vi "Scan Abort.vi"(8 "error in (no error)":errorcluster, 10 "Reference to a Stop button":refnum<vi>, 11 "VISA resource name":refnum<visa-resource-name>) -> (0 "error out":errorcluster, 3 "VISA resource name out":refnum<visa-resource-name>)   [LabVIEW 2009, in "Digikrom DK24x.lvlib"]
doc: "Inner loop that waits until scan completes or user pushes a specified abort button. Sends cancel command and stops all movement."
uses:
  Digikrom DK24x.lvlib
  Command.ctl
panel:
  in  "Manual Abort":bool
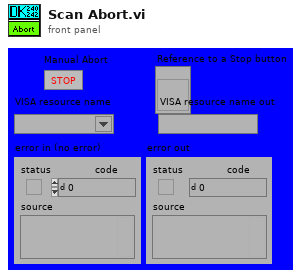
[diagram p1: front panel]
types:
  T1 = typedef "Digikrom DK24x.lvlib/Command.ctl" = u8
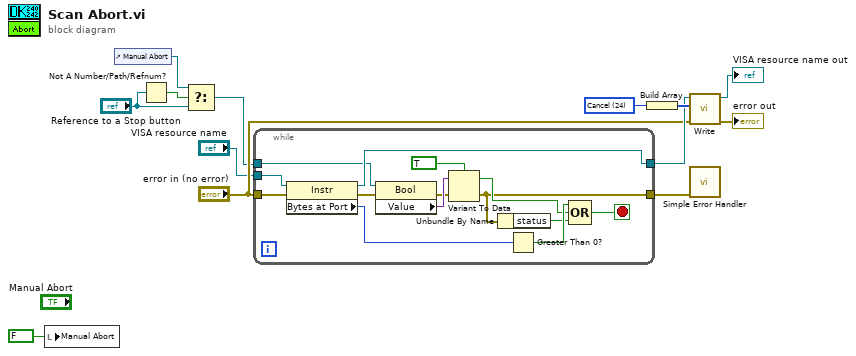
[diagram p0: block diagram]
diagram:
  w1 = T1 24 items=["Cancel"=24, "Clear"=25, "CSR"=28, "Echo"=27, "Filter"=15, "Gcal"=18, "Goto"=16, "Grtid?"=19, "Grtsel"=26, "NOVRAM Read"=56, "NOVRAM Write"=59, "Reset"=255, "Scan"=12, "Scan Up"=9, "Scan Down"=3, "Serial?"=33, "Slew Up"=8, "Slew Down"=2, "Slit Reset"=43, "Slit?"=30, "Sltadj"=14, "Speed"=13, "Sspeed?"=21, "Step Down"=1, "Step Up"=7, "S1adj"=31, "S2adj"=32, "S3adj"=34, "S1cal"=22, "S2cal"=23, "S3cal"=35, "Test"=17, "Type"=57, "Wave?"=29, "Zero"=52] ("Command")
  n1 = local write "Manual Abort"(FALSE ("Manual Abort")) -> ()
  n2 = control-ref of="Manual Abort"() -> (w6:refnum<vi>)
  n3 = Not A Number/Path/Refnum?(number/path/refnum="Reference to a Stop button") -> (NaN/Path/Refnum?=w4:bool)
  n4 = Select(t=w6, s=w4, f="Reference to a Stop button") -> (s? t:f=w3:refnum<vi>)
  n5 = while {
    tunnel: "error in (no error)" -> [w27]
    tunnel: "VISA resource name" -> [w25]
    tunnel: [w24] -> w12
    tunnel: [w16] -> w8
    tunnel: w3 -> [w14]
    stop <- w22 stop-if-true
    n6 = property class="Instr"(reference=w25, error in=w27) -> (reference out=w24:refnum<visa-resource-name>, error out=w26:errorcluster, "Bytes at Port"=w23:u32)
    n7 = property class="Bool"(reference=w14, error in=w26) -> (error out=w19:errorcluster, "Value"=w21:variant)  [unwired: 1 out]
    n8 = Variant To Data(error in=w19, Variant=w21, type=TRUE) -> (error out=w16:errorcluster, data=w17:bool)
    n9 = Unbundle By Name(w16) -> ("status"=w15:bool)
    n10 = Greater Than 0?(x=w23) -> (x > 0?=w18:bool)
    n11 = Compound Arithmetic op=OR(w18, w17, w15) -> (w22:bool)
  }
  n12 = Build Array(w1) -> (w13:T1[])
  n13 = call "Write.vi"("error in (no error)"="error in (no error)", "Byte Array"=w13, "VISA resource name"=w12) -> ("error out"=→"error out":errorcluster, "VISA resource name out"=→"VISA resource name out":refnum<visa-resource-name>)  [unwired: 7 out]
  n14 = call <vilib>:"Simple Error Handler.vi"("error in (no error)"=w8) -> ()  [unwired: 1 in, 8 out]
